vi "Build Graphs.vi"(9 "Start Time in Seconds":timestamp, 10 "Litho Point":T1, 11 "Reset Graphs":bool) -> (1 "Voltage":cluster{"X":dbl[], "Y":dbl[]}[](array[cluster]), 2 "Y Position":cluster{"X":dbl[], "Y":dbl[]}[](array[cluster]), 3 "X Position":cluster{"X":dbl[], "Y":dbl[]}[](array[cluster]))   [LabVIEW 2013]
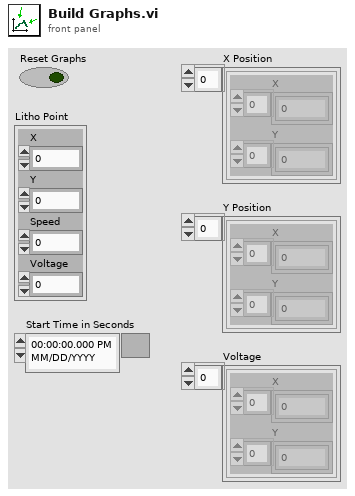
[diagram p1: front panel]
types:
  T1 = cluster{"X":dbl, "Y":dbl, "Speed":dbl, "Voltage":dbl}
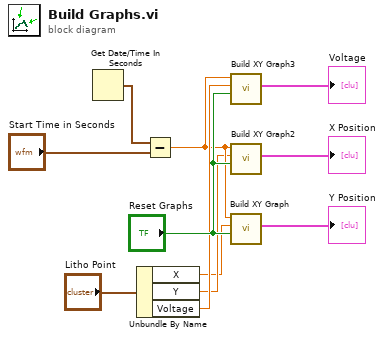
[diagram p0: block diagram]
diagram:
  n1 = Get Date/Time In Seconds() -> (seconds since 1Jan1904=w2:timestamp)
  n2 = Unbundle By Name("Litho Point") -> ("X"=w4:dbl, "Y"=w5:dbl, "Voltage"=w7:dbl)
  n3 = Subtract(x=w2, y="Start Time in Seconds") -> (x-y=w6:dbl)
  n4 = call "Build XY Graph3"("Reset"="Reset Graphs", "Y Input"=w7, "X Input"=w6) -> ("XY Graph"=→"Voltage":cluster{"X":dbl[], "Y":dbl[]}[])  [unwired: 7 in, 1 out]
  n5 = call "Build XY Graph2"("Reset"="Reset Graphs", "Y Input"=w5, "X Input"=w6) -> ("XY Graph"=→"X Position":cluster{"X":dbl[], "Y":dbl[]}[])  [unwired: 7 in, 1 out]
  n6 = call "Build XY Graph"("Reset"="Reset Graphs", "Y Input"=w4, "X Input"=w6) -> ("XY Graph"=→"Y Position":cluster{"X":dbl[], "Y":dbl[]}[])  [unwired: 7 in, 1 out]
